vi "Set Series CFG.vi"(8 "error in":errorcluster, 10 "Series CFG":string, 11 "Configuration UI Actor in":refnum<class "Configuration UI Actor.lvclass">) -> (0 "error out":errorcluster, 3 "Configuration UI Actor out":refnum<class "Configuration UI Actor.lvclass">)   [LabVIEW 2023, in "Configuration UI Actor.lvlib" / "Configuration UI Actor.lvclass"]
uses:
  Configuration UI Actor.lvclass
  Configuration UI Actor.lvclass/Configuration UI Actor.ctl
  <vilib>/JDP Science/JSONtext/JSONtext.lvlib
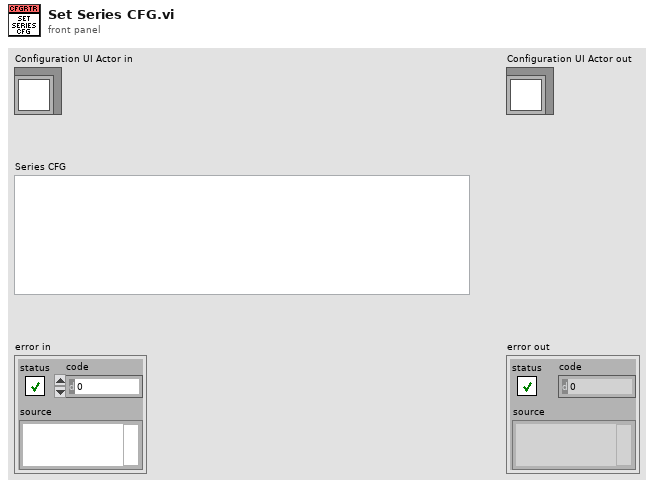
[diagram p1: front panel]
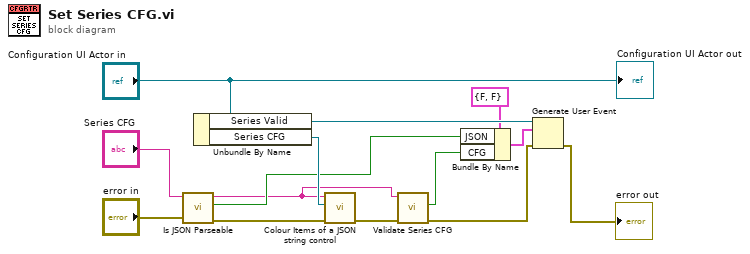
[diagram p0: block diagram]
diagram:
  n1 = call "Is JSON Parseable.vi"("error in (no error)"="error in", "<JSON>"="Series CFG") -> ("error out"=w13:errorcluster, "Valid?"=w9:bool, "Pretty <JSON>"=w7:string)  [unwired: 7 in]
  n2 = Unbundle By Name("Configuration UI Actor in") -> ("Series Valid"=w12:refnum<user-event>, "Series CFG"=w14:refnum<vi>)
  n3 = call <vilib>:"Colour Items of a JSON string control.vi"("error in (no error)"=w13, "String Control"=w14, "JSON"=w7) -> ("error out"=w8:errorcluster)  [unwired: 8 in]
  n4 = call "Validate Series CFG.vi"("error in"=w8, "<JSON>"=w7) -> ("error out"=w2:errorcluster, "Is Valid?"=w6:bool)  [unwired: 8 in]
  n5 = Bundle By Name(cluster=cluster{"JSON":bool, "CFG":bool} {"JSON"=FALSE, "CFG"=FALSE} ("Virt Valid"), "JSON"=w9, "CFG"=w6) -> (w10:cluster{"JSON":bool, "CFG":bool})
  n6 = Generate User Event(user event=w12, event data cluster=w10, error in=w2) -> (error out=→"error out":errorcluster)  [unwired: 1 in, 1 out]
  "Configuration UI Actor out" <- "Configuration UI Actor in"
